vi "test_F9P_fgv-ver.vi"() -> ()   [LabVIEW 2019] (continued)
25,11,294,,29,07,323,,6*60\r\n$GPGSV,4,4,13,30,01,134,,6*55\r\n$GLGSV,2,1,06,70,54,030,37,71,69,224,34,72,18,217,37,84,09,133,12,1*7D\r\n$GLGSV,2,2,06,85,63,111,41,86,51,337,,1*7F\r\n$GLGSV,2,1,06,70,54,030,,71,69,224,09,72,18,217,27,84,09,133,17,3*71\r\n$GLGSV,2,2,06,85,63,111,30,86,51,337,,3*7B\r\n$GAGSV,3,1,09,02,04,287,11,04,68,085,43,09,44,196,30,11,78,037,40,7*78\r\n$GAGSV,3,2,09,12,32,115,26,18,55,284,36,19,17,042,33,25,01,241,,7*73\r\n$GAGSV,3,3,09,36,35,314,33,7*4F\r\n$GAGSV,3,1,09,02,04,287,,04,68,085,36,09,44,196,30,11,78,037,32,2*7A\r\n$GAGSV,3,2,09,12,32,115,25,18,55,284,38,19,17,042,29,25,01,241,,2*70\r\n$GAGSV,3,3,09,36,35,314,24,2*4C\r\n$GBGSV,4,1,13,04,35,133,,05,09,257,,06,27,182,,07,09,201,,1*7B\r\n$GBGSV,4,2,13,08,65,355,40,09,07,194,,10,16,222,19,11,37,142,24,1*75\r\n$GBGSV,4,3,13,13,50,315,40,14,76,037,42,28,59,310,38,33,73,239,31,1*70\r\n$GBGSV,4,4,13,34,13,142,19,1*4E\r\n$GBGSV,4,1,13,04,35,133,,05,09,257,,06,27,182,,07,09,201,,3*79\r\n$GBGSV,4,2,13,08,65,355,37,09,07,194,,10,16,222,25,11,37,142,34,3*79\r\n$GBGSV,4,3,13,13,50,315,41,14,76,037,37,28,59,310,,33,73,239,,3*78\r\n$GBGSV,4,4,13,34,13,142,,3*44\r\n$GNGLL,3723.61684,N,12656.96898,E,064311.00,A,A*7E\r\n$GNRMC,064312.00,A,3723.61688,N,12656.96912,E,0.774,65.62,250720,,,A,V*3E\r\n$GNVTG,65.62,T,,M,0.774,N,1.433,K,A*15\r\n$GNGGA,064312.00,3723.61688,N,12656.96912,E,1,12,0.62,44.5,M,18.5,M,,*79\r\n$GNGSA,A,3,17,19,06,05,02,12,09,,,,,,1.09,0.62,0.90,1*01\r\n$GNGSA,A,3,85,70,71,72,,,,,,,,,1.09,0.62,0.90,2*0E\r\n$GNGSA,A,3,36,19,11,04,09,12,,,,,,,1.09,0.62,0.90,3*05\r\n$GNGSA,A,3,28,14,13,11,33,08,10,,,,,,1.09,0.62,0.90,4*05\r\n$GPGSV,4,1,13,02,65,334,43,04,08,037,39,05,48,261,36,06,58,076,47,1*63\r\n$GPGSV,4,2,13,07,06,105,,09,38,057,44,12,18,263,26,13,08,191,31,1*6D\r\n$GPGSV,4,3,13,17,19,158,23,19,37,161,25,25,11,294,,29,07,323,21,1*6A\r\n$GPGSV,4,4,13,30,01,134,,1*52\r\n$GPGSV,4,1,13,02,65,334,,04,08,037,34,05,48,261,33,06,58,076,38,6*63\r\n$GPGSV,4,2,13,07,06,105,,09,38,057,38,12,18,263,,13,08,191,,6*67\r\n$GPGSV,4,3,13,17,19,158,21,19,37,161,,25,11,294,,29,07,323,,6*6B\r\n$GPGSV,4,4,13,30,01,134,,6*55\r\n$GLGSV,2,1,06,70,54,030,30,71,69,224,30,72,18,217,31,84,09,133,13,1*79\r\n$GLGSV,2,2,06,85,63,111,41,86,51,337,,1*7F\r\n$GLGSV,2,1,06,70,54,030,,71,69,224,24,72,18,217,25,84,09,133,12,3*79\r\n$GLGSV,2,2,06,85,63,111,30,86,51,337,,3*7B\r\n$GAGSV,3,1,09,02,04,287,10,04,68,085,37,09,44,196,27,11,78,037,34,7*7F\r\n$GAGSV,3,2,09,12,32,115,31,18,55,284,36,19,17,042,33,25,01,241,,7*75\r\n$GAGSV,3,3,09,36,35,314,19,7*47\r\n$GAGSV,3,1,09,02,04,287,,04,68,085,31,09,44,196,24,11,78,037,33,2*79\r\n$GAGSV,3,2,09,12,32,115,32,18,55,284,35,19,17,042,,25,01,241,,2*70\r\n$GAGSV,3,3,09,36,35,314,22,2*4A\r\n$GBGSV,4,1,13,04,35,133,,05,09,257,,06,27,182,,07,09,201,,1*7B\r\n$GBGSV,4,2,13,08,65,355,40,09,07,194,,10,16,222,20,11,37,142,23,1*78\r\n$GBGSV,4,3,13,13,50,315,35,14,76,037,44,28,59,310,38,33,73,239,40,1*72\r\n$GBGSV,4,4,13,34,13,142,22,1*46\r\n$GBGSV,4,1,13,04,35,133,,05,09,257,,06,27,182,,07,09,201,,3*79\r\n$GBGSV,4,2,13,08,65,355,37,09,07,194,,10,16,222,22,11,37,142,26,3*7D\r\n$GBGSV,4,3,13,13,50,315,39,14,76,037,38,28,59,310,,33,73,239,,3*78\r\n$GBGSV,4,4,13,34,13,142,,3*44\r\n$GNGLL,3723.61688,N,12656.96912,E,064312.00,A,A*72\r\n$GNRMC,064313.00,A,3723.61693,N,12656.96917,E,0.197,,250720,,,A,V*12\r\n$GNVTG,,T,,M,0.197,N,0.366,K,A*31\r\n$GNGGA,064313.00,3723.61693,N,12656.96917,E,1,12,0.61,44.8,M,18.5,M,,*79\r\n$GNGSA,A,3,17,19,06,05,02,12,09,,,,,,1.06,0.61,0.87,1*0B\r\n$GNGSA,A,3,85,70,71,72,,,,,,,,,1.06,0.61,0.87,2*04\r\n$GNGSA,A,3,36,19,11,04,09,12,,,,,,,1.06,0.61,0.87,3*0F\r\n$GNGSA,A,3,28,34,14,13,11,33,08,10,,,,,1.06,0.61,0.87,4*08\r\n$GPGSV,4,1,13,02,65,334,43,04,08,037,41,05,48,261,40,06,58,076,39,1*64\r\n$GPGSV,4,2,13,07,06,105,,09,38,057,47,12,18,263,25,13,08,191,30,1*6C\r\n$GPGSV,4,3,13,17,19,158,30,19,37,161,31,25,11,294,,29,07,323,22,1*6E\r\n$GPGSV,4,4,13,30,01,134,,1*52\r\n$GPGSV,4,1,13,02,65,334,,04,08,037,37,05,48,261,33,06,58,076,40,6*6F\r\n$GPGSV,4,2,13,07,06,105,,09,38,057,41,12,18,263,,13,08,191,,6*69\r\n$GPGSV,4,3,13,17,19,158,20,19,37,161,,25,11,294,,29,07,323,,6*6A\r\n$GPGSV,4,4,13,30,01,134,,6*55\r\n$GLGSV,2,1,06,70,54,030,34,71,69,224,25,72,18,217,26,84,09,133,11,1*7D\r\n$GLGSV,2,2,06,85,63,111,36,86,51,337,,1*7F\r\n$GLGSV,2,1,06,70,54,030,,71,69,224,19,72,18,217,25,84,09,133,12,3*77\r\n$GLGSV,2,2,06,85,63,111,35,86,51,337,,3*7E\r\n$GAGSV,3,1,09,02,04,287,10,04,68,085,42,09,44,196,32,11,78,037,37,7*7A\r\n$GAGSV,3,2,09,12,32,115,37,18,55,284,38,19,17,042,33,25,01,241,,7*7D\r\n$GAGSV,3,3,09,36,35,314,28,7*45\r\n$GAGSV,3,1,09,02,04,287,,04,68,085,39,09,44,196,24,11,78,037,33,2*71\r\n$GAGSV,3,2,09,12,32,115,32,18,55,284,35,19,17,042,38,25,01,241,,2*7B\r\n$GAGSV,3,3,09,36,35,314,29,2*41\r\n$GBGSV,4,1,13,04,35,133,,05,09,257,,06,27,182,,07,09,201,,1*7B\r\n$GBGSV,4,2,13,08,65,355,41,09,07,194,,10,16,222,20,11,37,142,30,1*7B\r\n$GBGSV,4,3,13,13,50,315,41,14,76,037,42,28,59,310,42,33,73,239,38,1*75\r\n$GBGSV,4,4,13,34,13,142,23,1*47\r\n$GBGSV,4,1,13,04,35,133,,05,09,257,,06,27,182,,07,09,201,24,3*7F\r\n$GBGSV,4,2,13,08,65,355,39,09,07,194,,10,16,222,22,11,37,142,27,3*72\r\n$GBGSV,4,3,13,13,50,315,39,14,76,037,40,28,59,310,,33,73,239,,3*77\r\n$GBGSV,4,4,13,34,13,142,,3*44\r\n$GNGLL,3723.61693,N,12656.96917,E,064313.00,A,A*7C\r\n$GNRMC,064314.00,A,3723.61691,N,12656.96921,E,0.191,,250720,,,A,V*14\r\n$GNVTG,,T,,M,0.191,N,0.354,K,A*36\r\n$GNGGA,064314.00,3723.61691,N,12656.96921,E,1,12,0.62,45.1,M,18.5,M,,*72\r\n$GNGSA,A,3,17,19,06,05,02,12,09,,,,,,1.09,0.62,0.90,1*01\r\n$GNGSA,A,3,85,70,71,72,,,,,,,,,1.09,0.62,0.90,2*0E\r\n$GNGSA,A,3,36,19,11,04,09,12,,,,,,,1.09,0.62,0.90,3*05\r\n$GNGSA,A,3,28,14,13,11,33,08,10,,,,,,1.09,0.62,0.90,4*05\r\n$GPGSV,4,1,13,02,65,334,43,04,08,037,32,05,48,261,42,06,58,076,43,1*6F\r\n$GPGSV,4,2,13,07,06,105,,09,38,057,42,12,18,263,24,13,08,191,21,1*68\r\n$GPGSV,4,3,13,17,19,158,29,19,37,161,27,25,11,294,,29,07,323,20,1*63\r\n$GPGSV,4,4,13,30,01,134,,1*52\r\n$GPGSV,4,1,13,02,65,334,,04,08,037,40,05,48,261,36,06,58,076,28,6*64\r\n$GPGSV,4,2,13,07,06,105,,09,38,057,39,12,18,263,,13,08,191,,6*66\r\n$GPGSV,4,3,13,17,19,158,19,19,37,161,,25,11,294,,29,07,323,,6*60\r\n$GPGSV,4,4,13,30,01,134,,6*55\r\n$GLGSV,2,1,06,70,54,030,32,71,69,224,24,72,18,217,32,84,09,133,11,1*7F\r\n$GLGSV,2,2,06,85,63,111,32,86,51,337,,1*7B\r\n$GLGSV,2,1,06,70,54,030,,71,69,224,21,72,18,217,25,84,09,133,11,3*7F\r\n$GLGSV,2,2,06,85,63,111,32,86,51,337,,3*79\r\n$GAGSV,3,1,09,02,04,287,10,04,68,085,37,09,44,196,34,11,78,037,37,7*7E\r\n$GAGSV,3,2,09,12,32,115,24,18,55,284,43,19,17,042,28,25,01,241,,7*79\r\n$GAGSV,3,3,09,36,35,314,32,7*4E\r\n$GAGSV,3,1,09,02,04,287,,04,68,085,37,09,44,196,29,11,78,037,35,2*74\r\n$GAGSV,3,2,09,12,32,115,35,18,55,284,,19,17,042,29,25,01,241,,2*7A\r\n$GAGSV,3,3,09,36,35,314,29,2*41\r\n$GBGSV,4,1,13,04,35,133,,05,09,257,,06,27,182,,07,09,201,,1*7B\r\n$GBGSV,4,2,13,08,65,355,39,09,07,194,,10,16,222,22,11,37,142,29,1*7E\r\n$GBGSV,4,3,13,13,50,315,43,14,76,037,42,28,59,310,47,33,73,239,38,1*72\r\n$GBGSV,4,4,13,34,13,142,,1*46\r\n$GBGSV,4,1,13,04,35,133,,05,09,257,,06,27,182,,07,09,201,22,3*79\r\n$GBGSV,4,2,13,08,65,355,37,09,07,194,,10,16,222,20,11,37,142,32,3*7A\r\n$GBGSV,4,3,13,13,50,315,41,14,76,037,40,28,59,310,,33,73,239,,3*78\r\n$GBGSV,4,4,13,34,13,142,,3*44\r\n$GNGLL,3723.61691,N,12656.96921,E,064314.00,A,A*7C\r\n$GNRMC,064315.00,A,3723.61688,N,12656.96925,E,0.025,,250720,,,A,V*17\r\n$GNVTG,,T,,M,0.025,N,0.046,K,A*38\r\n$GNGGA,064315.00,3723.61688,N,12656.96925,E,1,12,0.70,45.2,M,18.5,M,,*7F\r\n$GNGSA,A,3,17,19,06,05,02,12,09,,,,,,1.30,0.70,1.09,1*09\r\n$GNGSA,A,3,85,70,71,72,,,,,,,,,1.30,0.70,1.09,2*06\r\n$GNGSA,A,3,36,19,11,04,09,12,,,,,,,1.30,0.70,1.09,3*0D\r\n$GNGSA,A,3,28,14,13,11,33,08,10,,,,,,1.30,0.70,1.09,4*0D\r\n$GPGSV,4,1,13,02,65,334,42,04,08,037,24,05,48,261,39,06,58,076,45,1*63\r\n$GPGSV,4,2,13,07,06,105,24,09,38,057,44,12,18,263,27,13,08,191,22,1*68\r\n$GPGSV,4,3,13,17,19,158,21,19,37,161,25,25,11,294,,29,07,323,21,1*68\r\n$GPGSV,4,4,13,30,01,134,,1*52\r\n$GPGSV,4,1,13,02,65,334,,04,08,037,33,05,48,261,38,06,58,076,35,6*62\r\n$GPGSV,4,2,13,07,06,105,,09,38,057,34,12,18,263,,13,08,191,,6*6B\r\n$GPGSV,4,3,13,17,19,158,19,19,37,161,,25,11,294,,29,07,323,,6*60\r\n$GPGSV,4,4,13,30,01,134,,6*55\r\n$GLGSV,2,1,06,70,54,030,34,71,69,224,31,72,18,217,38,84,09,133,09,1*7E\r\n$GLGSV,2,2,06,85,63,111,39,86,51,337,,1*70\r\n$GLGSV,2,1,06,70,54,030,,71,69,224,22,72,18,217,25,84,09,133,21,3*7F\r\n$GLGSV,2,2,06,85,63,111,30,86,51,337,,3*7B\r\n$GAGSV,3,1,09,02,04,287,07,04,68,085,39,09,44,196,29,11,78,037,38,7*75\r\n$GAGSV,3,2,09,12,32,115,24,18,55,284,41,19,17,042,26,25,01,241,,7*75\r\n$GAGSV,3,3,09,36,35,314,32,7*4E\r\n$GAGSV,3,1,09,02,04,287,,04,68,085,36,09,44,196,18,11,78,037,34,2*76\r\n$GAGSV,3,2,09,12,32,115,29,18,55,284,32,19,17,042,,25,01,241,,2*7D\r\n$GAGSV,3,3,09,36,35,314,31,2*48\r\n$GBGSV,4,1,13,04,35,133,,05,09,257,,06,27,182,,07,09,201,,1*7B\r\n$GBGSV,4,2,13,08,65,355,40,09,07,194,,10,16,222,22,11,37,142,23,1*7A\r\n$GBGSV,4,3,13,13,50,315,42,14,76,037,42,28,59,310,45,33,73,239,42,1*7C\r\n$GBGSV,4,4,13,34,13,142,,1*46\r\n$GBGSV,4,1,13,04,35,133,,05,09,257,,06,27,182,,07,09,201,21,3*7A\r\n$GBGSV,4,2,13,08,65,355,38,09,07,194,,10,16,222,19,11,37,142,30,3*7D\r\n$GBGSV,4,3,13,13,50,315,35,14,76,037,39,28,59,310,,33,73,239,,3*75\r\n$GBGSV,4,4,13,34,13,142,,3*44\r\n$GNGLL,3723.61688,N,12656.96925,E,064315.00,A,A*71\r\n$GNRMC,064316.00,A,3723.61692,N,12656.96928,E,0.287,,250720,,,A,V*18\r\n$GNVTG,,T,,M,0.287,N,0.531,K,A*37\r\n$GNGGA,064316.00,3723.61692,N,12656.96928,E,1,12,0.67,45.1,M,18.5,M,,*7F\r\n$GNGSA,A,3,17,19,06,05,02,12,09,,,,,,1.19,0.67,0.98,1*0D\r\n$GNGSA,A,3,85,70,71,72,,,,,,,,,1.19,0.67,0.98,2*02\r\n$GNGSA,A,3,36,19,11,04,09,12,,,,,,,1.19,0.67,0.98,3*09\r\n$GNGSA,A,3,28,14,13,11,33,08,10,,,,,,1.19,0.67,0.98,4*09\r\n$GPGSV,4,1,13,02,65,334,45,04,08,037,40,05,48,261,25,06,58,076,40,1*6E\r\n$GPGSV,4,2,13,07,06,105,,09,38,057,31,12,18,263,26,13,08,191,29,1*66\r\n$GPGSV,4,3,13,17,19,158,29,19,37,161,31,25,11,294,,29,07,323,21,1*65\r\n$GPGSV,4,4,13,30,01,134,,1*52\r\n$GPGSV,4,1,13,02,65,334,,04,08,037,22,05,48,261,32,06,58,076,30,6*6D\r\n$GPGSV,4,2,13,07,06,105,,09,38,057,21,12,18,263,,13,08,191,,6*6F\r\n$GPGSV,4,3,13,17,19,158,18,19,37,161,,25,11,294,,29,07,323,,6*61\r\n$GPGSV,4,4,13,30,01,134,,6*55\r\n$GLGSV,2,1,06,70,54,030,31,71,69,224,35,72,18,217,29,84,09,133,09,1*7F\r\n$GLGSV,2,2,06,85,63,111,41,86,51,337,,1*7F\r\n$GLGSV,2,1,06,70,54,030,,71,69,224,29,72,18,217,25,84,09,133,17,3*71\r\n$GLGSV,2,2,06,85,63,111,33,86,51,337,,3*78\r\n$GAGSV,3,1,09,02,04,287,07,04,68,085,39,09,44,196,28,11,78,037,38,7*74\r\n$GAGSV,3,2,09,12,32,115,23,18,55,284,38,19,17,042,30,25,01,241,,7*7B\r\n$GAGSV,3,3,09,36,35,314,31,7*4D\r\n$GAGSV,3,1,09,02,04,287,,04,68,085,35,09,44,196,20,11,78,037,31,2*7B\r\n$GAGSV,3,2,09,12,32,115,30,18,55,284,26,19,17,042,,25,01,241,,2*70\r\n$GAGSV,3,3,09,36,35,314,30,2*49\r\n$GBGSV,4,1,13,04,35,133,,05,09,257,,06,27,182,,07,09,201,,1*7B\r\n$GBGSV,4,2,13,08,65,355,40,09,07,194,,10,16,222,22,11,37,142,26,1*7F\r\n$GBGSV,4,3,13,13,50,315,41,14,76,037,39,28,59,310,44,33,73,239,38,1*7F\r\n$GBGSV,4,4,13,34,13,142,,1*46\r\n$GBGSV,4,1,13,04,35,133,,05,09,257,,06,27,182,,07,09,201,20,3*7B\r\n$GBGSV,4,2,13,08,65,355,36,09,07,194,,10,16,222,18,11,37,142,25,3*76\r\n$GBGSV,4,3,13,13,50,315,41,14,76,037,29,28,59,310,,33,73,239,,3*77\r\n$GBGSV,4,4,13,34,13,142,,3*44\r\n$GNGLL,3723.61692,N,12656.96928,E,064316.00,A,A*74\r\n$GNRMC,064317.00,A,3723.61674,N,12656.96912,E,1.140,169.59,250720,,,A,V*0D\r\n$GNVTG,169.59,T,,M,1.140,N,2.111,K,A*26\r\n$GNGGA,064317.00,3723.61674,N,12656.96912,E,1,12,0.62,44.6,M,18.5,M,,*7C\r\n$GNGSA,A,3,17,19,06,05,02,12,09,,,,,,1.09,0.62,0.90,1*01\r\n$GNGSA,A,3,85,70,71,72,,,,,,,,,1.09,0.62,0.90,2*0E\r\n$GNGSA,A,3,36,19,11,04,09,12,,,,,,,1.09,0.62,0.90,3*05\r\n$GNGSA,A,3,28,14,13,11,33,08,10,,,,,,1.09,0.62,0.90,4*05\r\n$GPGSV,4,1,13,02,65,334,44,04,08,037,35,05,48,261,37,06,58,076,46,1*68\r\n$GPGSV,4,2,13,07,06,105,,09,38,057,45,12,18,263,25,13,08,191,29,1*66\r\n$GPGSV,4,3,13,17,19,158,28,19,37,161,31,25,11,294,08,29,07,323,20,1*6D\r\n$GPGSV,4,4,13,30,01,134,,1*52\r\n$GPGSV,4,1,13,02,65,334,,04,08,037,31,05,48,261,31,06,58,076,31,6*6D\r\n$GPGSV,4,2,13,07,06,105,,09,38,057,37,12,18,263,,13,08,191,,6*68\r\n$GPGSV,4,3,13,17,19,158,20,19,37,161,,25,11,294,,29,07,323,,6*6A\r\n$GPGSV,4,4,13,30,01,134,,6*55\r\n$GLGSV,2,1,06,70,54,030,32,71,69,224,27,72,18,217,33,84,09,133,08,1*75\r\n$GLGSV,2,2,06,85,63,111,43,86,51,337,,1*7D\r\n$GLGSV,2,1,06,70,54,030,,71,69,224,27,72,18,217,25,84,09,133,18,3*70\r\n$GLGSV,2,2,06,85,63,111,21,86,51,337,,3*7B\r\n$GAGSV,3,1,09,02,04,287,11,04,68,085,43,09,44,196,32,11,78,037,42,7*78\r\n$GAGSV,3,2,09,12,32,115,29,18,55,284,30,19,17,042,31,25,01,241,,7*78\r\n$GAGSV,3,3,09,36,35,314,24,7*49\r\n$GAGSV,3,1,09,02,04,287,,04,68,085,35,09,44,196,23,11,78,037,35,2*7C\r\n$GAGSV,3,2,09,12,32,115,30,18,55,284,35,19,17,042,,25,01,241,,2*72\r\n$GAGSV,3,3,09,36,35,314,28,2*40\r\n$GBGSV,4,1,13,04,35,133,,05,09,257,,06,27,182,,07,09,201,,1*7B\r\n$GBGSV,4,2,13,08,65,355,40,09,07,194,,10,16,222,21,11,37,142,28,1*72\r\n$GBGSV,4,3,13,13,50,315,37,14,76,037,44,28,59,310,40,33,73,239,35,1*7D\r\n$GBGSV,4,4,13,34,13,142,,1*46\r\n$GBGSV,4,1,13,04,35,133,,05,09,257,,06,27,182,,07,09,201,21,3*7A\r\n$GBGSV,4,2,13,08,65,355,35,09,07,194,,10,16,222,19,11,37,142,,3*73\r\n$GBGSV,4,3,13,13,50,315,40,14,76,037,40,28,59,310,,33,73,239,,3*79\r\n$GBGSV,4,4,13,34,13,142,,3*44\r\n$GNGLL,3723.61674,N,12656.96912,E,064317.00,A,A*74\r\n$GNRMC,064318.00,A,3723.61665,N,12656.96904,E,0.169,,250720,,,A,V*13\r\n$GNVTG,,T,,M,0.169,N,0.314,K,A*35\r\n$GNGGA,064318.00,3723.61665,N,12656.96904,E,1,12,0.66,44.3,M,18.5,M,,*75\r\n$GNGSA,A,3,17,19,06,05,02,09,,,,,,,1.18,0.66,0.98,1*0E\r\n$GNGSA,A,3,85,70,71,72,,,,,,,,,1.18,0.66,0.98,2*02\r\n$GNGSA,A,3,36,19,11,04,09,12,,,,,,,1.18,0.66,0.98,3*09\r\n$GNGSA,A,3,28,14,13,11,33,08,10,,,,,,1.18,0.66,0.98,4*09\r\n$GPGSV,4,1,13,02,65,334,46,04,08,037,38,05,48,261,30,06,58,076,44,1*62\r\n$GPGSV,4,2,13,07,06,105,,09,38,057,42,12,18,263,,13,08,191,18,1*64\r\n$GPGSV,4,3,13,17,19,158,22,19,37,161,22,25,11,294,09,29,07,323,20,1*64\r\n$GPGSV,4,4,13,30,01,134,,1*52\r\n$GPGSV,4,1,13,02,65,334,,04,08,037,25,05,48,261,32,06,58,076,35,6*6F\r\n$GPGSV,4,2,13,07,06,105,,09,38,057,42,12,18,263,,13,08,191,,6*6A\r\n$GPGSV,4,3,13,17,19,158,19,19,37,161,,25,11,294,,29,07,323,,6*60\r\n$GPGSV,4,4,13,30,01,134,,6*55\r\n$GLGSV,2,1,06,70,54,030,32,71,69,224,25,72,18,217,37,84,08,134,08,1*75\r\n$GLGSV,2,2,06,85,63,111,38,86,51,337,,1*71\r\n$GLGSV,2,1,06,70,54,030,,71,69,224,24,72,18,217,25,84,08,134,15,3*78\r\n$GLGSV,2,2,06,85,63,111,32,86,51,337,,3*79\r\n$GAGSV,3,1,09,02,04,287,07,04,68,085,41,09,44,196,35,11,78,037,41,7*79\r\n$GAGSV,3,2,09,12,32,115,29,18,55,284,27,19,17,042,37,25,01,241,,7*78\r\n$GAGSV,3,3,09,36,35,314,30,7*4C\r\n$GAGSV,3,1,09,02,04,287,,04,68,085,38,09,44,196,31,11,78,037,31,2*76\r\n$GAGSV,3,2,09,12,32,115,32,18,55,284,35,19,17,042,,25,01,241,,2*70\r\n$GAGSV,3,3,09,36,35,314,24,2*4C\r\n$GBGSV,4,1,13,04,35,133,,05,09,257,,06,27,182,,07,09,201,,1*7B\r\n$GBGSV,4,2,13,08,65,355,41,09,07,194,,10,16,222,20,11,37,142,25,1*7F\r\n$GBGSV,4,3,13,13,50,315,40,14,76,037,41,28,59,310,40,33,73,239,26,1*7A\r\n$GBGSV,4,4,13,34,13,142,,1*46\r\n$GBGSV,4,1,13,04,35,133,,05,09,257,,06,27,182,,07,09,201,20,3*7B\r\n$GBGSV,4,2,13,08,65,355,34,09,07,194,,10,16,222,21,11,37,142,,3*79\r\n$GBGSV,4,3,13,13,50,315,40,14,76,037,35,28,59,310,,33,73,239,,3*7B\r\n$GBGSV,4,4,13,34,13,142,,3*44\r\n$GNGLL,3723.61665,N,12656.96904,E,064318.00,A,A*7C\r\n$GNRMC,064319.00,A,3723.61665,N,12656.96906,E,0.068,,250720,,,A,V*10\r\n$GNVTG,,T,,M,0.068,N,0.125,K,A*35\r\n$GNGGA,064319.00,3723.61665,N,12656.96906,E,1,12,0.66,44.3,M,18.5,M,,*76\r\n$GNGSA,A,3,17,19,06,05,02,12,09,,,,,,1.18,0.66,0.98,1*0D\r\n$GNGSA,A,3,85,70,71,72,,,,,,,,,1.18,0.66,0.98,2*02\r\n$GNGSA,A,3,36,19,11,04,09,12,,,,,,,1.18,0.66,0.98,3*09\r\n$GNGSA,A,3,28,14,13,11,33,08,10,,,,,,1.18,0.66,0.98,4*09\r\n$GPGSV,4,1,13,02,65,334,46,04,08,037,35,05,48,261,18,06,58,076,44,1*65\r\n$GPGSV,4,2,13,07,06,105,,09,38,057,43,12,18,263,27,13,08,191,21,1*6A\r\n$GPGSV,4,3,13,17,19,158,24,19,37,161,30,25,11,294,12,29,07,323,21,1*6A\r\n$GPGSV,4,4,13,30,01,134,,1*52\r\n$GPGSV,4,1,13,02,65,334,,04,08,037,22,05,48,261,32,06,58,076,30,6*6D\r\n$GPGSV,4,2,13,07,06,105,,09,38,057,41,12,18,263,,13,08,191,,6*69\r\n$GPGSV,4,3,13,17,19,158,20,19,37,161,,25,11,294,,29,07,323,,6*6A\r\n$GPGSV,4,4,13,30,01,134,,6*55\r\n$GLGSV,2,1,06,70,54,030,33,71,69,224,32,72,18,217,34,84,08,134,13,1*7B\r\n$GLGSV,2,2,06,85,63,113,37,86,51,337,,1*7C\r\n$GLGSV,2,1,06,70,54,030,,71,69,224,21,72,18,217,26,84,08,134,18,3*73\r\n$GLGSV,2,2,06,85,63,113,26,86,51,337,,3*7E\r\n$GAGSV,3,1,09,02,04,287,10,04,68,085,38,09,44,196,30,11,78,037,39,7*7B\r\n$GAGSV,3,2,09,12,32,115,31,18,55,284,28,19,17,042,22,25,01,241,,7*7A\r\n$GAGSV,3,3,09,36,35,314,32,7*4E\r\n$GAGSV,3,1,09,02,04,287,,04,68,085,35,09,44,196,32,11,78,037,30,2*79\r\n$GAGSV,3,2,09,12,32,115,29,18,55,284,38,19,17,042,,25,01,241,,2*77\r\n$GAGSV,3,3,09,36,35,314,25,2*4D\r\n$GBGSV,4,1,13,04,35,133,,05,09,257,,06,27,182,,07,09,201,,1*7B\r\n$GBGSV,4,2,13,08,65,355,41,09,07,194,,10,16,222,20,11,37,142,21,1*7B\r\n$GBGSV,4,3,13,13,50,315,41,14,76,037,40,28,59,310,43,33,73,239,28,1*77\r\n$GBGSV,4,4,13,34,13,142,,1*46\r\n$GBGSV,4,1,13,04,35,133,,05,09,257,,06,27,182,,07,09,201,18,3*70\r\n$GBGSV,4,2,13,08,65,355,34,09,07,194,,10,16,222,25,11,37,142,,3*7D\r\n$GBGSV,4,3,13,13,50,315,40,14,76,037,29,28,59,310,,33,73,239,,3*76\r\n$GBGSV,4,4,13,34,13,142,,3*44\r\n$GNGLL,3723.61665,N,12656.96906,E,064319.00,A,A*7F\r\n$GNRMC,064320.00,A,3723.61671,N,12656.96908,E,0.079,,250720,,,A,V*11\r\n$GNVTG,,T,,M,0.079,N,0.147,K,A*31\r\n$GNGGA,064320.00,3723.61671,N,12656.96908,E,1,12,0.65,44.5,M,18.5,M,,*72\r\n$GNGSA,A,3,17,19,06,05,02,12,09,,,,,,1.13,0.65,0.93,1*0E\r\n$GNGSA,A,3,85,70,71,72,,,,,,,,,1.13,0.65,0.93,2*01\r\n$GNGSA,A,3,36,19,11,04,09,12,,,,,,,1.13,0.65,0.93,3*0A\r\n$GNGSA,A,3,28,14,13,33,08,10,,,,,,,1.13,0.65,0.93,4*0A\r\n$GPGSV,4,1,13,02,65,334,44,04,08,037,35,05,48,261,21,06,58,076,42,1*6B\r\n$GPGSV,4,2,13,07,06,105,26,09,38,057,43,12,18,263,27,13,08,191,21,1*6E\r\n$GPGSV,4,3,13,17,19,158,24,19,37,161,23,25,11,294,13,29,07,323,20,1*68\r\n$GPGSV,4,4,13,30,01,134,,1*52\r\n$GPGSV,4,1,13,02,65,334,,04,08,037,18,05,48,261,30,06,58,076,32,6*64\r\n$GPGSV,4,2,13,07,06,105,,09,38,057,39,12,18,263,,13,08,191,,6*66\r\n$GPGSV,4,3,13,17,19,158,22,19,37,161,,25,11,294,,29,07,323,,6*68\r\n$GPGSV,4,4,13,30,01,134,,6*55\r\n$GLGSV,2,1,06,70,54,030,35,71,69,224,31,72,18,217,35,84,08,134,11,1*7D\r\n$GLGSV,2,2,06,85,63,113,37,86,52,337,,1*7F\r\n$GLGSV,2,1,06,70,54,030,,71,69,224,16,72,18,217,26,84,08,134,17,3*78\r\n$GLGSV,2,2,06,85,63,113,26,86,52,337,,3*7D\r\n$GAGSV,3,1,09,02,04,287,08,04,68,085,38,09,44,196,30,11,78,037,39,7*72\r\n$GAGSV,3,2,09,12,32,115,32,18,55,284,29,19,17,042,20,25,01,241,,7*7A\r\n$GAGSV,3,3,09,36,35,314,34,7*48\r\n$GAGSV,3,1,09,02,04,287,,04,68,085,36,09,44,196,33,11,78,037,29,2*73\r\n$GAGSV,3,2,09,12,32,115,28,18,55,284,37,19,17,042,33,25,01,241,,2*79\r\n$GAGSV,3,3,09,36,35,314,24,2*4C\r\n$GBGSV,4,1,13,04,35,133,,05,09,257,,06,27,182,,07,09,201,,1*7B\r\n$GBGSV,4,2,13,08,65,355,41,09,07,194,,10,16,222,20,11,37,142,,1*78\r\n$GBGSV,4,3,13,13,50,315,42,14,76,037,40,28,59,310,44,33,73,239,26,1*7D\r\n$GBGSV,4,4,13,34,13,142,,1*46\r\n$GBGSV,4,1,13,04,35,133,,05,09,257,,06,27,182,,07,09,201,16,3*7E\r\n$GBGSV,4,2,13,08,65,355,34,09,07,194,,10,16,222,27,11,37,142,,3*7F\r\n$GBGSV,4,3,13,13,50,315,40,14,76,037,30,28,59,310,,33,73,239,,3*7E\r\n$GBGSV,4,4,13,34,13,142,,3*44\r\n$GNGLL,3723.61671,N,12656.96908,E,064320.00,A,A*7E\r\n$GNRMC,064321.00,A,3723.61676,N,12656.96910,E,0.046,,250720,,,A,V*12\r\n$GNVTG,,T,,M,0.046,N,0.085,K,A*32\r\n$GNGGA,064321.00,3723.61676,N,12656.96910,E,1,12,0.62,44.5,M,18.5,M,,*7A\r\n$GNGSA,A,3,17,19,06,05,02,12,09,,,,,,1.09,0.62,0.90,1*01\r\n$GNGSA,A,3,85,70,71,72,,,,,,,,,1.09,0.62,0.90,2*0E\r\n$GNGSA,A,3,36,19,11,04,09,12,,,,,,,1.09,0.62,0.90,
